vi "Send Fwd Message to Nested Actor.vi"(0 "Message Enqueuer":refnum<class "Message Enqueuer.lvclass">, 1 "Message Priority (Normal)":T2=enum."Normal", 5 "Entity Type":T1, 7 "Entity Index":i32, 9 "Message":refnum<class "Message.lvclass">, 11 "error in (no error)":errorcluster) -> (4 "Message Enqueuer out":refnum<class "Message Enqueuer.lvclass">, 15 "error out":errorcluster)   [LabVIEW 2023, in "Coffee Shop.lvlib" / "Fwd Message to Nested Actor Msg.lvclass"]
doc: "This VI sends the message to an actor."
uses:
  Fwd Message to Nested Actor Msg.lvclass
  <vilib>/ActorFramework/Message Enqueuer/Message Enqueuer.lvclass
  <vilib>/ActorFramework/Message Enqueuer/Message Priority.ctl
  Coffee Shop/Entity Types.ctl
  <vilib>/ActorFramework/Message/Message.lvclass
  c:/dev/_r/4/eng/lv-core/lvpostprocessingd/lv_mc_x86_64/dist_i386/vi.lib/ActorFramework/Message/Message.lvclass
  Fwd Message to Nested Actor Msg.lvclass/Fwd Message to Nested Actor Msg.ctl
  <vilib>/ActorFramework/Message Enqueuer/Message Enqueuer.lvclass/Message Enqueuer.ctl
  <vilib>/ActorFramework/Message Priority Queue/Priority Enqueue.vi
  Coffee Shop/Coffee Shop.lvclass
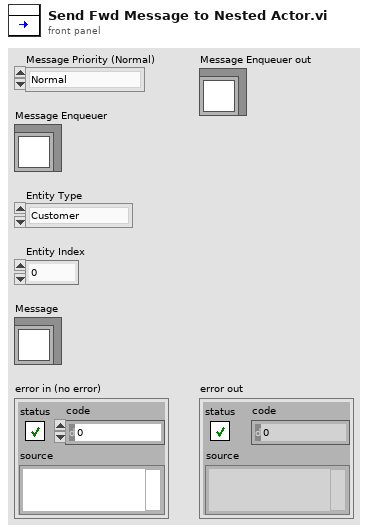
[diagram p1: front panel]
types:
  T1 = typedef "Coffee Shop.lvlib/Coffee Shop.lvclass/Entity Types.ctl" = enum16{"Customer", "Cashier", "Barista"}
  T2 = typedef "Actor Framework.lvlib/Message Enqueuer.lvclass/Message Priority.ctl" = enum16{"Low", "Normal", "High"}
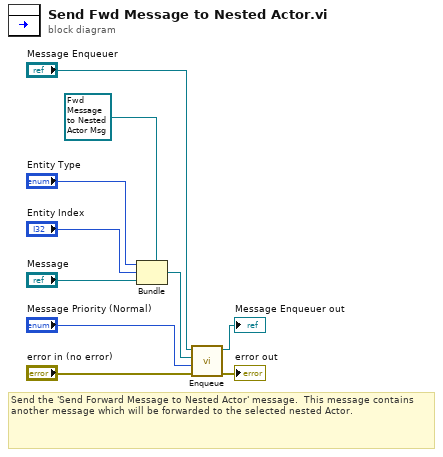
[diagram p0: block diagram]
diagram:
  # "Send the 'Send Forward Message to Nested Actor' message.  This message contains another message which will be forwarded to the selected nested Actor."
  n1 = Bundle(cluster=refnum<class "Fwd Message to Nested Actor Msg.lvclass"> refnum ("Object"), "Entity Type", "Entity Index", "Message") -> (w6:refnum<class "Fwd Message to Nested Actor Msg.lvclass">)
  n2 = call <vilib>:"Enqueue.vi"("error in (no error)"="error in (no error)", "Message Priority (Normal)"="Message Priority (Normal)", "Message"=w6, "Message Enqueuer in"="Message Enqueuer") -> ("error out"=→"error out":errorcluster, "Message Enqueuer out"=→"Message Enqueuer out":refnum<class "Message Enqueuer.lvclass">)  [unwired: 6 in]
